vi "Define_Indicies_Connect_Points_Subtracks(111_as_101)-2.vi"(3 "error IN":errorcluster, 4 "[IN] Index of single track\n(problem displacement)":i32, 5 "[IN] Index of problem\ndisplacement inside track":i32, 6 "[IN] Track group":T1) -> (0 "error OUT":errorcluster, 1 "[OUT] Index of \nconnected dots\ninside the track":i32[](array[numeric]), 2 "[OUT] Index of connected\ntracks with problem dot":i32[](array[numeric]))   [LabVIEW 2013]
doc: "The subVI scans subtracks for defining connected with input problem point"
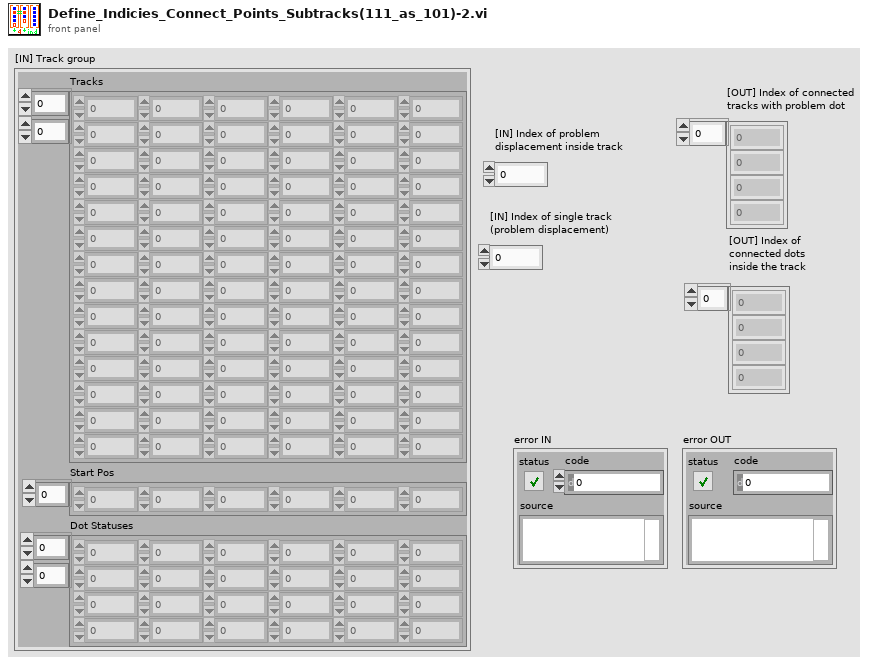
[diagram p1: front panel]
types:
  T1 = cluster{"Tracks":dbl[][], "Start Pos":i32[], "Dot Statuses":i16[][]}
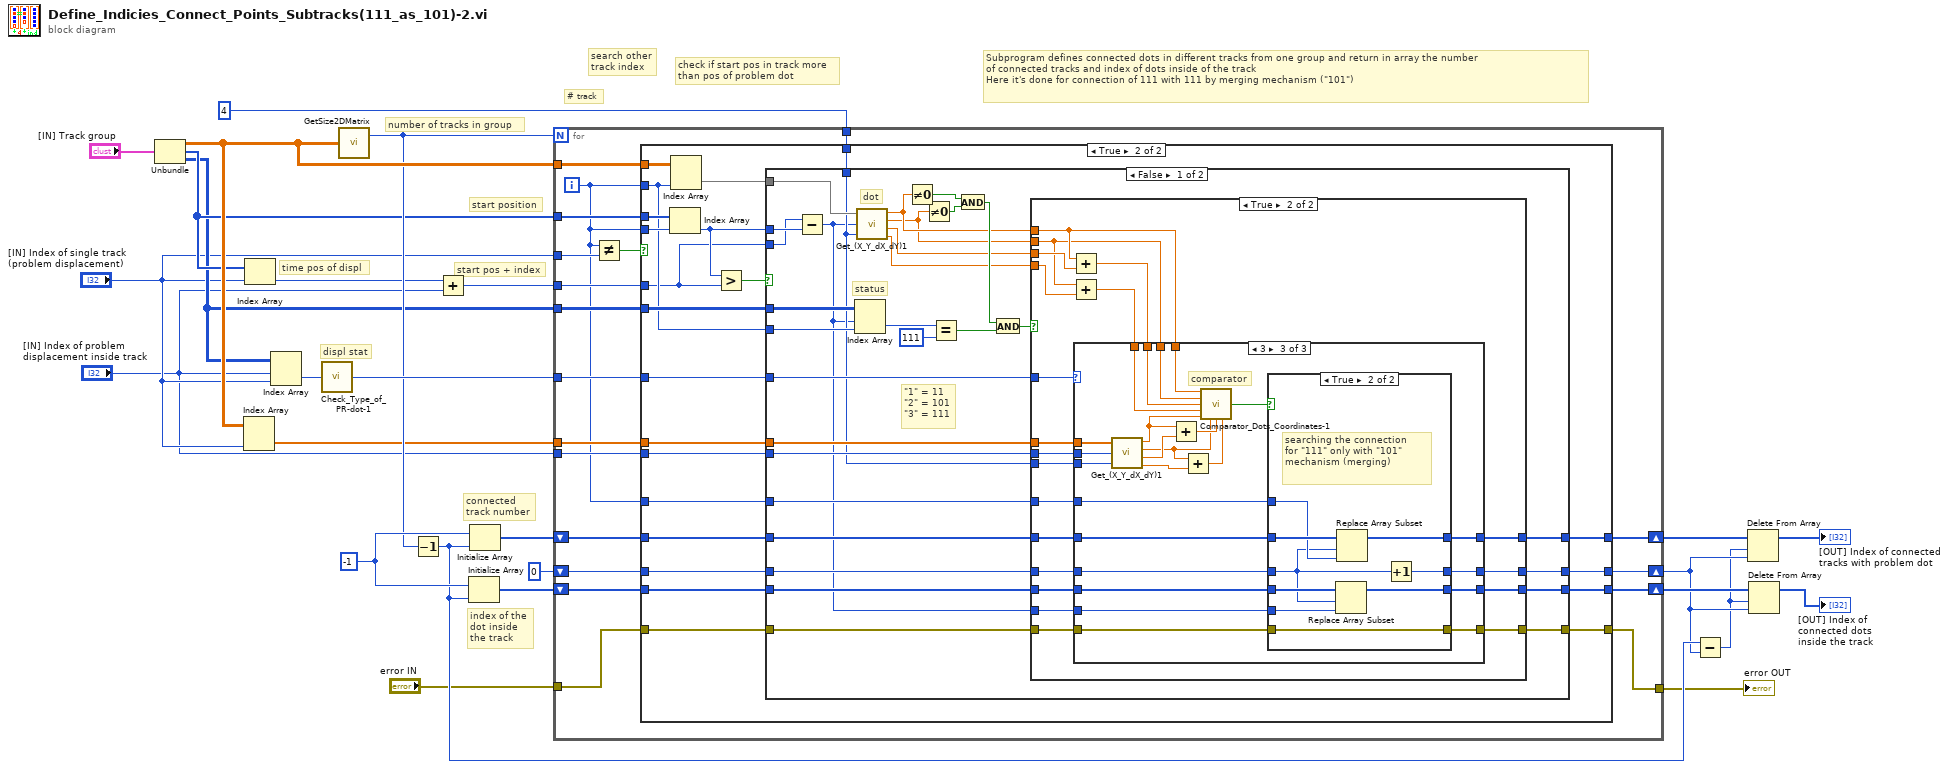
[diagram p0: block diagram]
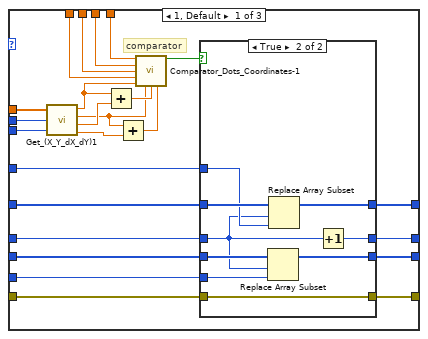
[diagram p4: hidden frame]
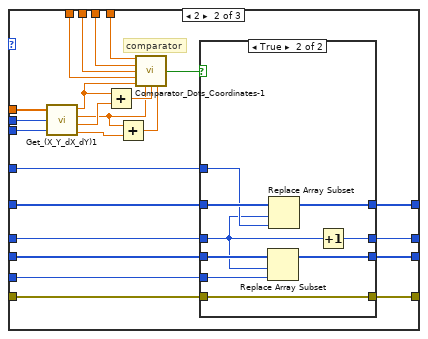
[diagram p6: hidden frame]
diagram:
  w22 = -1 ("disabled index (row)")
  # "start pos + index"
  # "Subprogram defines connected dots in different tracks from one group and return in array the number\nof connected tracks and index of dots inside of the track\nHere it's done for connection of 111 with 111 by merging mechanism (\"101\")"
  # "# track"
  # "start position"
  # "number of tracks in group"
  # "check if start pos in track more \nthan pos of problem dot"
  # "search other\ntrack index"
  # "time pos of displ"
  # "index of the dot inside \nthe track"
  # "connected\ntrack number"
  # "displ stat"
  n1 = Unbundle("[IN] Track group") -> ("Tracks"=w24:dbl[][], "Start Pos"=w17:i32[], "Dot Statuses"=w15:i16[][])
  n2 = Index Array(array=w24, index (col)="[IN] Index of single track\n(problem displacement)") -> (element=w14:dbl[])  [unwired: 1 in]
  n3 = Index Array(array=w17, index="[IN] Index of single track\n(problem displacement)") -> (element=w2:i32)
  n4 = Index Array(array=w15, index (row)="[IN] Index of problem\ndisplacement inside track", index (col)="[IN] Index of single track\n(problem displacement)") -> (element=w25:i16)
  n5 = call "Check_Type_of_PR-dot-1.vi"("[IN] dot status"=w25) -> ("[OUT] Type of\nproblem dot"=w23:i32)
  n6 = call "GetSize2DMatrix.vi"("Array IN (2D)"=w24) -> ("# Cols"=w21:i32)  [unwired: 1 out]
  n7 = Decrement(x=w21) -> (x-1=w12:i32)
  n8 = Add(x=w2, y="[IN] Index of problem\ndisplacement inside track") -> (x+y=w4:i32)
  n9 = Initialize Array(w22, w12) -> (w19:i32[])
  n10 = Initialize Array(w22, w12) -> (w20:i32[])
  n11 = for {
    N: w21 -> [_]
    tunnel: w24 -> [w43]
    tunnel: w23 -> [w39]
    tunnel: w4 -> [w40]
    shift-right: [w31] -> w13
    shift-left: w20 -> [w42]
    shift-right: [w29] -> w11
    shift-left: w19 -> [w41]
    tunnel: "[IN] Index of single track\n(problem displacement)" -> [w45]
    shift-right: [w30] -> w10
    shift-left: 0 -> [w38]
    tunnel: w17 -> [w37]
    tunnel: 4 ("multiplier") -> [w36]
    tunnel: w15 -> [w35]
    tunnel: w14 -> [w34]
    tunnel: "[IN] Index of problem\ndisplacement inside track" -> [w33]
    tunnel: "error IN" -> [w28]
    tunnel: [w27] -> w5
    i -> [w32]
    n12 = Not Equal?(x=w32, y=w45) -> (x != y?=w44:bool)
    n13 = case shown="True" w44 {
      tunnel: w43 -> [_ w71]
      tunnel: w32 -> [_ w63]
      tunnel: w42 -> [w49 w59]
      tunnel: w41 -> [w47 w57]
      tunnel: w40 -> [_ w50]
      tunnel: w39 -> [_ w62]
      tunnel: w38 -> [w48 w58]
      tunnel: w37 -> [_ w70]
      tunnel: w32 -> [_ w69]
      tunnel: w36 -> [_ w65]
      tunnel: w35 -> [_ w64]
      tunnel: w34 -> [_ w61]
      tunnel: w33 -> [_ w60]
      tunnel: w32 -> [_ w56]
      tunnel: [w49 w55] -> w31
      tunnel: [w48 w54] -> w30
      tunnel: [w47 w53] -> w29
      tunnel: w28 -> [w46 w52]
      tunnel: [w46 w51] -> w27
      frame False {
      }
      frame True {
        n14 = Index Array(array=w70, index=w69) -> (element=w66:i32)
        n15 = Index Array(array=w71, index (col)=w63) -> (element=w67:dbl[])  [unwired: 1 in]
        n16 = Greater?(x=w66, y=w50) -> (0:w68:bool)
        n17 = case shown="False" w68 {
          tunnel: w67 -> [w101 _]
          tunnel: w66 -> [w100 _]
          tunnel: w50 -> [w99 _]
          tunnel: w65 -> [w82 _]
          tunnel: w64 -> [w96 _]
          tunnel: w63 -> [w95 _]
          tunnel: w62 -> [w89 _]
          tunnel: w61 -> [w84 _]
          tunnel: w60 -> [w83 _]
          tunnel: w59 -> [w81 w240]
          tunnel: w58 -> [w80 w239]
          tunnel: w57 -> [w79 w238]
          tunnel: w56 -> [w78 _]
          tunnel: [w76 w240] -> w55
          tunnel: [w75 w239] -> w54
          tunnel: [w74 w238] -> w53
          tunnel: w52 -> [w73 w237]
          tunnel: [w72 w237] -> w51
          frame False {
            # "\"1\" = 11\n\"2\" = 101\n\"3\" = 111"
            # "status"
            # "dot"
            n18 = Subtract(x=w99, y=w100) -> (x-y=w77:i32)
            n19 = Index Array(array=w96, index (row)=w77, index (col)=w95) -> (element=w94:i16)
            n20 = call "Get_(X_Y_dX_dY)1.vi"("(X,Y,dX,dY)"=w101, "index"=w77, "multiplier"=w82) -> ("X"=w88:dbl, "Y"=w87:dbl, "dX"=w86:dbl, "dY"=w85:dbl)
            n21 = Not Equal To 0?(x=w88) -> (x != 0?=w97:bool)
            n22 = Not Equal To 0?(x=w87) -> (x != 0?=w98:bool)
            n23 = Equal?(x=w94, y=i16 111) -> (x = y?=w91:bool)
            n24 = And(x=w97, y=w98) -> (x .and. y?=w92:bool)
            n25 = And(x=w92, y=w91) -> (x .and. y?=w90:bool)
            n26 = case shown="True" w90 {
              tunnel: w89 -> [_ w125]
              tunnel: w88 -> [_ w119]
              tunnel: w87 -> [_ w118]
              tunnel: w86 -> [_ w121]
              tunnel: w85 -> [_ w120]
              tunnel: w84 -> [_ w124]
              tunnel: w83 -> [_ w123]
              tunnel: w82 -> [_ w122]
              tunnel: w81 -> [w105 w115]
              tunnel: w80 -> [w104 w114]
              tunnel: w79 -> [w103 w113]
              tunnel: w78 -> [_ w112]
              tunnel: w77 -> [_ w111]
              tunnel: [w105 w110] -> w76
              tunnel: [w104 w109] -> w75
              tunnel: [w103 w108] -> w74
              tunnel: w73 -> [w102 w107]
              tunnel: [w102 w106] -> w72
              frame False {
              }
              frame True {
                n27 = Add(x=w119, y=w121) -> (x+y=w117:dbl)
                n28 = Add(x=w118, y=w120) -> (x+y=w116:dbl)
                n29 = case shown="3" w125 {
                  tunnel: w124 -> [w149 w176 w217]
                  tunnel: w123 -> [w148 w175 w216]
                  tunnel: w122 -> [w147 w174 w215]
                  tunnel: w119 -> [w146 w177 w211]
                  tunnel: w118 -> [w145 w178 w212]
                  tunnel: w117 -> [w144 w179 w213]
                  tunnel: w116 -> [w143 w180 w214]
                  tunnel: w115 -> [w135 w171 w209]
                  tunnel: w114 -> [w134 w170 w208]
                  tunnel: w113 -> [w133 w169 w207]
                  tunnel: w112 -> [w132 w172 w210]
                  tunnel: w111 -> [w131 w168 w206]
                  tunnel: [w130 w167 w205] -> w110
                  tunnel: [w129 w166 w204] -> w109
                  tunnel: [w128 w165 w203] -> w108
                  tunnel: w107 -> [w127 w164 w202]
                  tunnel: [w126 w163 w201] -> w106
                  frame 1, Default {
                    # "comparator"
                    n30 = call "Get_(X_Y_dX_dY)1.vi"("(X,Y,dX,dY)"=w149, "index"=w148, "multiplier"=w147) -> ("X"=w142:dbl, "Y"=w139:dbl, "dX"=w141:dbl, "dY"=w138:dbl)
                    n31 = Add(x=w142, y=w141) -> (x+y=w140:dbl)
                    n32 = Add(x=w139, y=w138) -> (x+y=w137:dbl)
                    n33 = call "Comparator_Dots_Coordinates-1.vi"("X1"=w146, "Y1"=w145, "(X+dX)1"=w144, "(Y+dY)1"=w143, "X2"=w142, "Y2"=w139, "(X+dX)2"=w140, "(Y+dY)2"=w137) -> ("X1=X2,Y1=Y2 (1)"=w136:bool)  [unwired: 5 in, 2 out]
                    n34 = case shown="True" w136 {
                      tunnel: w135 -> [w153 w162]
                      tunnel: w134 -> [w152 w158]
                      tunnel: w133 -> [w151 w160]
                      tunnel: w132 -> [_ w161]
                      tunnel: w131 -> [_ w159]
                      tunnel: [w153 w157] -> w130
                      tunnel: [w152 w156] -> w129
                      tunnel: [w151 w155] -> w128
                      tunnel: [w150 w154] -> w126
                      tunnel: w127 -> [w150 w154]
                      frame False {
                      }
                      frame True {
                        n35 = Replace Array Subset(array=w160, new element=w159, index=w158) -> (w155:i32[])
                        n36 = Replace Array Subset(array=w162, new element=w161, index=w158) -> (w157:i32[])
                        n37 = Increment(x=w158) -> (x+1=w156:i32)
                      }
                    }
                  }
                  frame 2 {
                    # "comparator"
                    n38 = call "Get_(X_Y_dX_dY)1.vi"("(X,Y,dX,dY)"=w176, "index"=w175, "multiplier"=w174) -> ("X"=w186:dbl, "Y"=w183:dbl, "dX"=w185:dbl, "dY"=w182:dbl)
                    n39 = Add(x=w186, y=w185) -> (x+y=w184:dbl)
                    n40 = Add(x=w183, y=w182) -> (x+y=w181:dbl)
                    n41 = call "Comparator_Dots_Coordinates-1.vi"("X1"=w177, "Y1"=w178, "(X+dX)1"=w179, "(Y+dY)1"=w180, "X2"=w186, "Y2"=w183, "(X+dX)2"=w184, "(Y+dY)2"=w181) -> ("X1(2)=X2(2),Y1(2)=Y2(2) (2)"=w173:bool)  [unwired: 5 in, 2 out]
                    n42 = case shown="True" w173 {
                      tunnel: w171 -> [w190 w199]
                      tunnel: w170 -> [w189 w195]
                      tunnel: w169 -> [w188 w197]
                      tunnel: w172 -> [_ w198]
                      tunnel: w168 -> [_ w196]
                      tunnel: [w190 w194] -> w167
                      tunnel: [w189 w193] -> w166
                      tunnel: [w188 w192] -> w165
                      tunnel: w164 -> [w187 w191]
                      tunnel: [w187 w191] -> w163
                      frame False {
                      }
                      frame True {
                        n43 = Replace Array Subset(array=w197, new element=w196, index=w195) -> (w192:i32[])
                        n44 = Replace Array Subset(array=w199, new element=w198, index=w195) -> (w194:i32[])
                        n45 = Increment(x=w195) -> (x+1=w193:i32)
                      }
                    }
                  }
                  frame 3 {
                    # "comparator"
                    n46 = call "Get_(X_Y_dX_dY)1.vi"("(X,Y,dX,dY)"=w217, "index"=w216, "multiplier"=w215) -> ("X"=w223:dbl, "Y"=w220:dbl, "dX"=w222:dbl, "dY"=w219:dbl)
                    n47 = Add(x=w223, y=w222) -> (x+y=w221:dbl)
                    n48 = Add(x=w220, y=w219) -> (x+y=w218:dbl)
                    n49 = call "Comparator_Dots_Coordinates-1.vi"("X1"=w211, "Y1"=w212, "(X+dX)1"=w213, "(Y+dY)1"=w214, "X2"=w223, "Y2"=w220, "(X+dX)2"=w221, "(Y+dY)2"=w218) -> ("X1(2)=X2(2),Y1(2)=Y2(2) (2)"=w200:bool)  [unwired: 5 in, 2 out]
                    n50 = case shown="True" w200 {
                      tunnel: w209 -> [w227 w236]
                      tunnel: w208 -> [w226 w232]
                      tunnel: w207 -> [w225 w234]
                      tunnel: w210 -> [_ w235]
                      tunnel: w206 -> [_ w233]
                      tunnel: [w227 w231] -> w205
                      tunnel: [w226 w230] -> w204
                      tunnel: [w225 w229] -> w203
                      tunnel: w202 -> [w224 w228]
                      tunnel: [w224 w228] -> w201
                      frame False {
                      }
                      frame True {
                        # "searching the connection\nfor \"111\" only with \"101\"\nmechanism (merging)"
                        n51 = Replace Array Subset(array=w234, new element=w233, index=w232) -> (w229:i32[])
                        n52 = Replace Array Subset(array=w236, new element=w235, index=w232) -> (w231:i32[])
                        n53 = Increment(x=w232) -> (x+1=w230:i32)
                      }
                    }
                  }
                }
              }
            }
          }
          frame True {
          }
        }
      }
    }
  }
  "error OUT" <- w5
  n54 = Subtract(x=w12, y=w10) -> (x-y=w9:i32)
  n55 = Delete From Array(array=w13, length=w9, index=w10) -> (array with subset deleted=→"[OUT] Index of connected\ntracks with problem dot":i32[])  [unwired: 1 out]
  n56 = Delete From Array(array=w11, length=w9, index=w10) -> (array with subset deleted=→"[OUT] Index of \nconnected dots\ninside the track":i32[])  [unwired: 1 out]
